vi "pelletron_query.vi"(8 "error in (no error)":errorcluster, 10 "Lower Timestamp Limit":i64, 11 "Upper Timestamp Limit":i64=3) -> (0 "error out":errorcluster, 3 "Pelletron Data":T1[](array[typedef]))   [LabVIEW 2013]
doc: "Selects rows from pelletron_data by timestamp."
uses:
  Controls/Pelletron.ctl
  <vilib>/addons/database/_DB Variant To Data/Database Variant To Data.xnode
panel:
  out "SQL Query Syntax":string
  # "Pelletron"
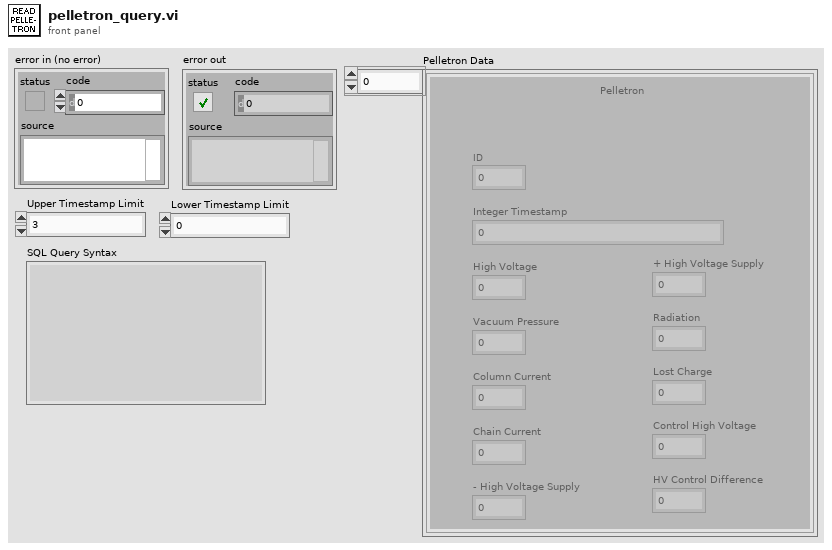
[diagram p1: front panel]
types:
  T1 = typedef "Pelletron.ctl" = cluster{"ID":i32, "Integer Timestamp":u64, "High Voltage":sgl, "+ High Voltage Supply":sgl, "- High Voltage Supply":sgl, "HV Control Difference":sgl, "Vacuum Pressure":sgl, "Radiation":sgl, "Column Current":sgl, "Lost Charge":sgl, "Chain Current":sgl, "Control High Voltage":sgl}
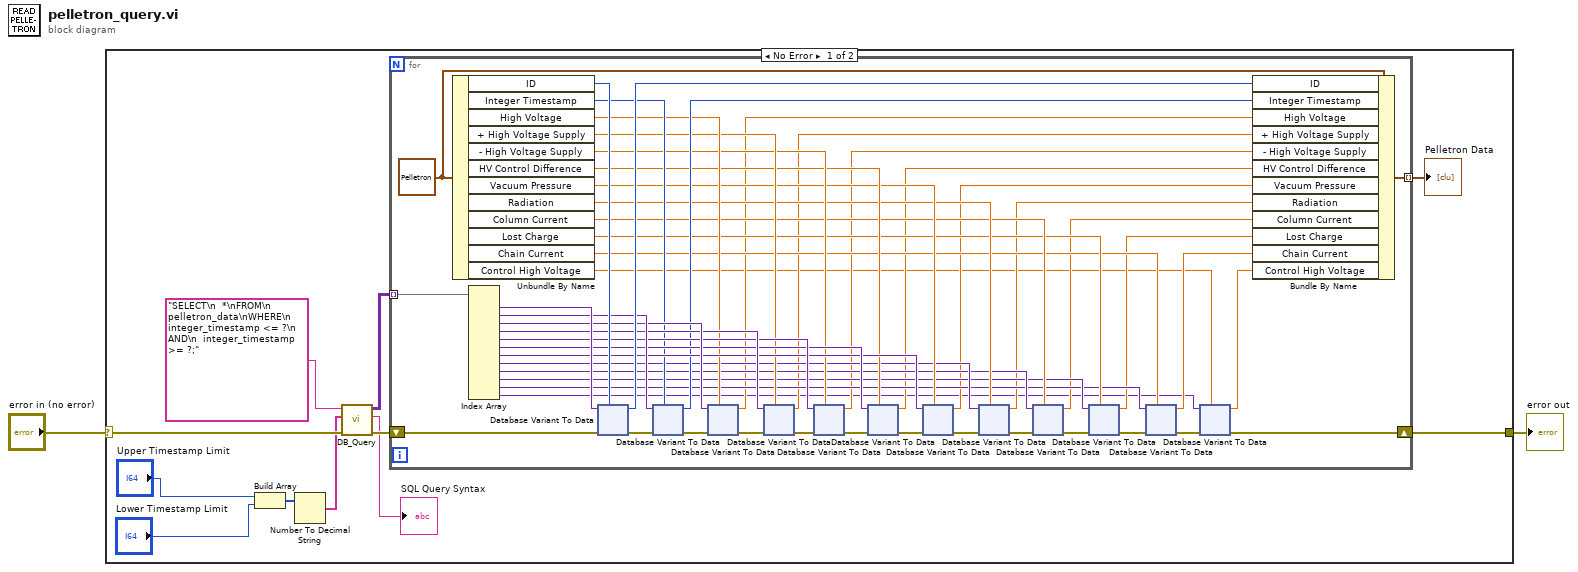
[diagram p0: block diagram]
diagram:
  n1 = case shown="No Error" "error in (no error)" {
    selector: "error in (no error)" -> [w11 w450]
    tunnel: [w12 w450] -> w1
    frame No Error {
      n2 = Build Array("Upper Timestamp Limit", "Lower Timestamp Limit") -> (w7:i64[])
      n3 = Number To Decimal String(number=w7) -> (decimal integer string=w6:string[])  [unwired: 1 in]
      n4 = call "DB_Query.vi"("error in (no error)"=w11, "Parameters"=w6, "Parameterized Query"="SELECT\n  *\nFROM\n  pelletron_data\nWHERE\n  integer_timestamp <= ?\n    AND\n  integer_timestamp >= ?;" ("string")) -> ("error out"=w10:errorcluster, "Query in Standard Format"=→"SQL Query Syntax":string, "Results"=w3:variant[][])  [unwired: 6 in]
      n5 = for {
        tunnel: [w21] -> w13 mode=indexing
        shift-right: [w14] -> w12
        shift-left: w10 -> [w20]
        tunnel: w3 -> [w19] mode=indexing
        w65 = T1 {"ID"=0, "Integer Timestamp"=0, "High Voltage"=0.0, "+ High Voltage Supply"=0.0, "- High Voltage Supply"=0.0, "HV Control Difference"=0.0, "Vacuum Pressure"=0.0, "Radiation"=0.0, "Column Current"=0.0, "Lost Charge"=0.0, "Chain Current"=0.0, "Control High Voltage"=0.0} ("Cluster")
        n6 = Unbundle By Name(w65) -> ("ID"=w64:i32, "Integer Timestamp"=w54:u64, "High Voltage"=w53:sgl, "+ High Voltage Supply"=w52:sgl, "- High Voltage Supply"=w51:sgl, "HV Control Difference"=w50:sgl, "Vacuum Pressure"=w49:sgl, "Radiation"=w48:sgl, "Column Current"=w47:sgl, "Lost Charge"=w46:sgl, "Chain Current"=w45:sgl, "Control High Voltage"=w17:sgl)
        n7 = Index Array(array=w19) -> (element #1=w62:variant, element #2=w61:variant, element #3=w60:variant, element #4=w59:variant, element #5=w58:variant, element #6=w57:variant, element #7=w56:variant, element #8=w44:variant, element #9=w43:variant, element #10=w42:variant, element #11=w41:variant, element #12=w16:variant)  [unwired: 12 in]
        n8 = xnode "Database Variant To Data"("database variant"=w62, "error in (no error)"=w20, "type"=w64) -> ("data"=w63:i32, "error out"=w31:errorcluster)
        n9 = xnode "Database Variant To Data"("database variant"=w61, "error in (no error)"=w31, "type"=w54) -> ("data"=w55:u64, "error out"=w30:errorcluster)
        n10 = xnode "Database Variant To Data"("database variant"=w60, "error in (no error)"=w30, "type"=w53) -> ("data"=w40:sgl, "error out"=w29:errorcluster)
        n11 = xnode "Database Variant To Data"("database variant"=w59, "error in (no error)"=w29, "type"=w52) -> ("data"=w39:sgl, "error out"=w28:errorcluster)
        n12 = xnode "Database Variant To Data"("database variant"=w58, "error in (no error)"=w28, "type"=w51) -> ("data"=w38:sgl, "error out"=w27:errorcluster)
        n13 = xnode "Database Variant To Data"("database variant"=w57, "error in (no error)"=w27, "type"=w50) -> ("data"=w37:sgl, "error out"=w26:errorcluster)
        n14 = xnode "Database Variant To Data"("database variant"=w56, "error in (no error)"=w26, "type"=w49) -> ("data"=w36:sgl, "error out"=w25:errorcluster)
        n15 = xnode "Database Variant To Data"("database variant"=w44, "error in (no error)"=w25, "type"=w48) -> ("data"=w35:sgl, "error out"=w24:errorcluster)
        n16 = xnode "Database Variant To Data"("database variant"=w43, "error in (no error)"=w24, "type"=w47) -> ("data"=w34:sgl, "error out"=w23:errorcluster)
        n17 = xnode "Database Variant To Data"("database variant"=w42, "error in (no error)"=w23, "type"=w46) -> ("data"=w33:sgl, "error out"=w22:errorcluster)
        n18 = xnode "Database Variant To Data"("database variant"=w41, "error in (no error)"=w22, "type"=w45) -> ("data"=w32:sgl, "error out"=w18:errorcluster)
        n19 = xnode "Database Variant To Data"("database variant"=w16, "error in (no error)"=w18, "type"=w17) -> ("data"=w15:sgl, "error out"=w14:errorcluster)
        n20 = Bundle By Name(cluster=w65, "ID"=w63, "Integer Timestamp"=w55, "High Voltage"=w40, "+ High Voltage Supply"=w39, "- High Voltage Supply"=w38, "HV Control Difference"=w37, "Vacuum Pressure"=w36, "Radiation"=w35, "Column Current"=w34, "Lost Charge"=w33, "Chain Current"=w32, "Control High Voltage"=w15) -> (w21:T1)
      }
      "Pelletron Data" <- w13
    }
    frame Error {
    }
  }
  "error out" <- w1
